vi "Accelerometer Logic.vi"(3 "Sensitivity":i8, 5 "Acceleration":dbl(slide) scale=-1.0..1.0) -> (2 "Position":dbl)   [LabVIEW 2014]
panel:
  out "Velocity":dbl
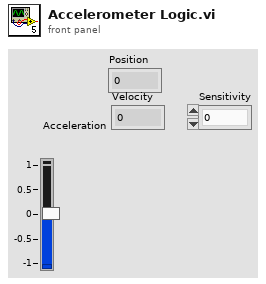
[diagram p1: front panel]
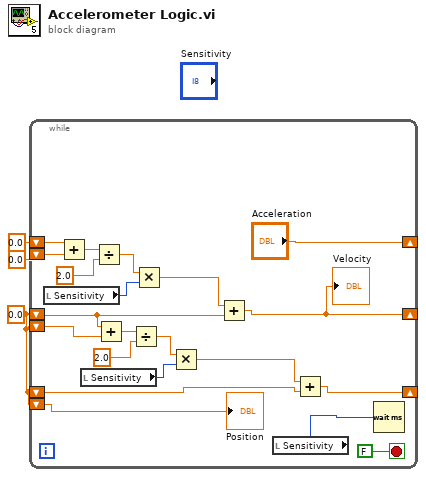
[diagram p0: block diagram]
diagram:
  w1 = 0.0
  n1 = while {
    shift-right: ["Acceleration"] -> _
    shift-left: 0.0 ("X-Axis") -> [w19]
    shift-left: 0.0 ("X-Axis") -> [w20]
    shift-right: [w22] -> _
    shift-left: w1 -> [w9]
    shift-left: w1 -> [w8]
    shift-right: [w7] -> _
    shift-left: w1 -> [w5]
    shift-left: w1 -> [w4]
    stop <- FALSE stop-if-true
    n2 = local read "Sensitivity"() -> (w15:i8)
    n3 = Add(x=w19, y=w20) -> (x+y=w18:dbl)
    n4 = local read "Sensitivity"() -> (w13:i8)
    n5 = Divide(x=w18, y=2.0) -> (x/y=w16:dbl)
    n6 = Add(x=w9, y=w8) -> (x+y=w10:dbl)
    n7 = Divide(x=w10, y=2.0) -> (x/y=w12:dbl)
    n8 = Multiply(x=w16, y=w15) -> (x*y=w14:dbl)
    n9 = Multiply(x=w12, y=w13) -> (x*y=w6:dbl)
    n10 = Add(x=w14, y=w9) -> (x+y=w22:dbl)
    "Velocity" <- w22
    n11 = local read "Sensitivity"() -> (w21:i8)
    n12 = Add(x=w6, y=w5) -> (x+y=w7:dbl)
    n13 = Wait (ms)(milliseconds to wait=w21) -> ()  [unwired: 1 out]
    "Position" <- w4
  }
